vi "Image Folder.vi"(11 "Main VI path":path) -> (3 "Image Folder path":path)   [LabVIEW 2018]
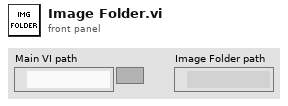
[diagram p1: front panel]
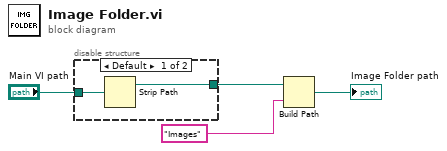
[diagram p0: block diagram]
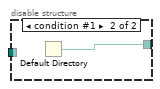
[diagram p2: hidden frame]
diagram:
  n1 = disable-structure shown="Default" {
    disable-tunnel: "Main VI path" -> [w6 _]
    disable-tunnel: [w5 w7] -> w4
    frame condition #0 (active) {
      n2 = Strip Path(path=w6) -> (stripped path=w5:path)  [unwired: 1 out]
    }
    frame condition #1 {
      n3 = Default Directory() -> (w7:path)
    }
  }
  n4 = Build Path(base path=w4, name or relative path="Images") -> (appended path=→"Image Folder path":path)
